vi "Autonomous Independent.vi"() -> ()   [LabVIEW 2012]
doc: "This VI is called when autonomous begins, and will automatically be terminated when autonomous ends. You can carry out timed or sensor driven robot movement independently without needing to return to the caller."
uses:
  Robot Global Data.vi
panel:
  out "Current Movement, for debugging":T1 {"Y Joystick Value" scale=1.0..-1.0; "X Joystick Value" scale=-1.0..1.0}
  in  "Array of robot movements":T2(array[cluster]) {"Y Joystick Value" scale=1.0..-1.0; "X Joystick Value" scale=-1.0..1.0}
  # "Be sure to right-click and choose Data Operations>>Make Current Value default if you want to save the array values with the VI"
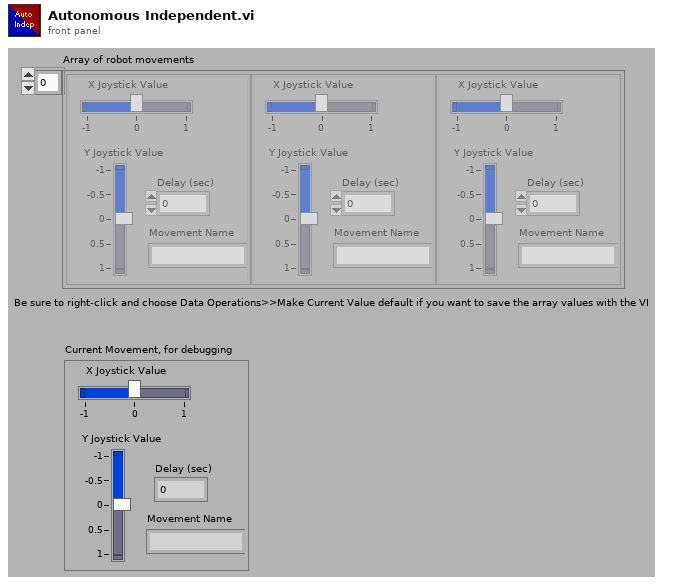
[diagram p1: front panel]
types:
  T1 = cluster{"X Joystick Value":dbl, "Y Joystick Value":dbl, "Delay (sec)":dbl, "Movement Name":string}
  T2 = cluster{"X Joystick Value":dbl, "Y Joystick Value":dbl, "Delay (sec)":dbl, "Movement Name":string}[]
  T3 = typedef "WPI_JoystickDevRef.ctl" = cluster{"Device":T4}
  T4 = typedef "WPI_JoystickDeviceEnum.ctl" = enum16{"USB 1", "USB 2", "USB 3", "USB 4", "Kinect 1", "Kinect 2"}
  T5 = cluster{"axis 1 (x)":dbl, "axis 2 (y)":dbl, "axis 3 (throttle)":dbl, "axis 4":dbl, "axis 5":dbl, "axis 6":dbl}
  T6 = typedef "WPI_DigitalInputDevRef.ctl" = cluster{"DevStatus":errorcluster, "DIO Channel":T7, "Digital Module":T8}
  T7 = typedef "FPGA_DIOChannel.ctl" = enum8{"DIO 1", "DIO 2", "DIO 3", "DIO 4", "DIO 5", "DIO 6", "DIO 7", "DIO 8", "DIO 9", "DIO 10", "DIO 11", "DIO 12", "DIO 13", "DIO 14", "Invalid"}
  T8 = typedef "FPGA_TypedefDigitalModule.ctl" = enum16{"Digital Module 1", "Digital Module 2"}
  T9 = typedef "WPI_RobotDriveDevRef.ctl" = cluster{"DevStatus":errorcluster, "Motors[]":T10[], "Square Inputs":bool, "Max Output":dbl, "Isochronous":bool}
  T10 = typedef "WPI_MotorControlDeviceRef.ctl" = cluster{"DeviceStatus":errorcluster, "Type":enum16{"PWM", "CAN"}, "PWM":cluster{"Digital Module":T8, "PWM Channel":T11, "DeadBand":T12}, "CAN":cluster{"Device Number":u8, "Control Mode":T13, "Semaphore":T14, "Max Vout":dbl}, "Invert":bool, "TransformRef":T15, "InvTransformRef":T15}
  T11 = typedef "FPGA_DIOPWMChannel.ctl" = enum8{"PWM 1", "PWM 2", "PWM 3", "PWM 4", "PWM 5", "PWM 6", "PWM 7", "PWM 8", "PWM 9", "PWM 10", "Invalid"}
  T12 = typedef "WPI_PWMDeadband.ctl" = cluster{"Name":string, "maxPositivePwm":i32, "minPositivePwm":i32, "centerPwm":i32, "maxNegativePwm":i32, "minNegativePwm":i32, "angularRange":u16}
  T13 = typedef "WPI_CANJaguar_ControlMode.ctl" = enum8{"Percent VBus", "Current", "Speed", "Position", "Voltage"}
  T14 = typedef "Semaphore RefNum" = refnum<k1>
  T15 = typedef "WPI_PWMTransform_ConPane.ctl" = refnum<vi>
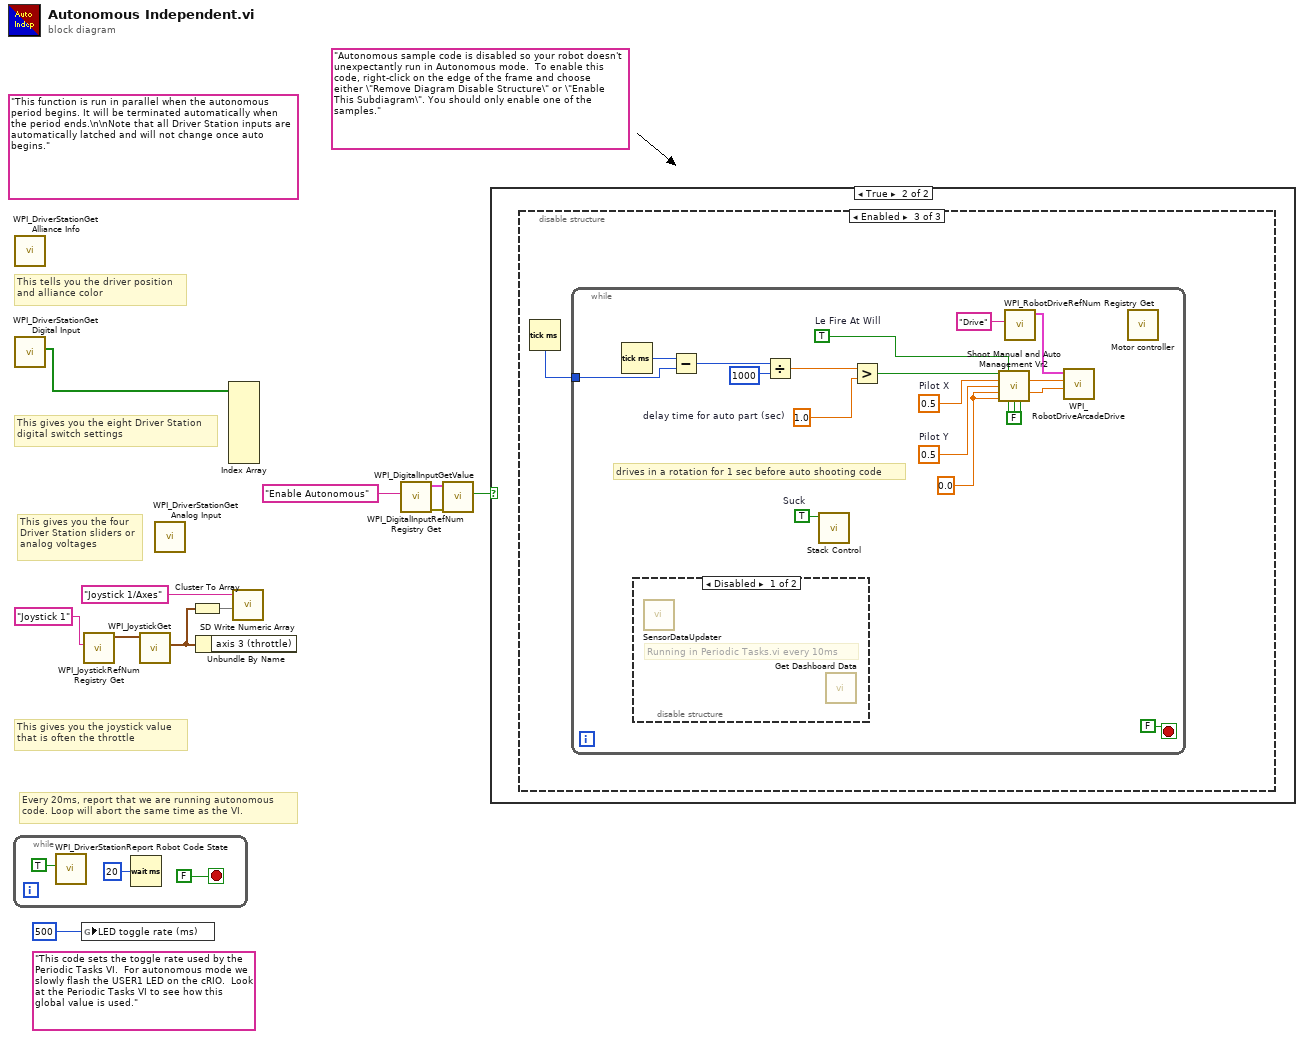
[diagram p0: block diagram]
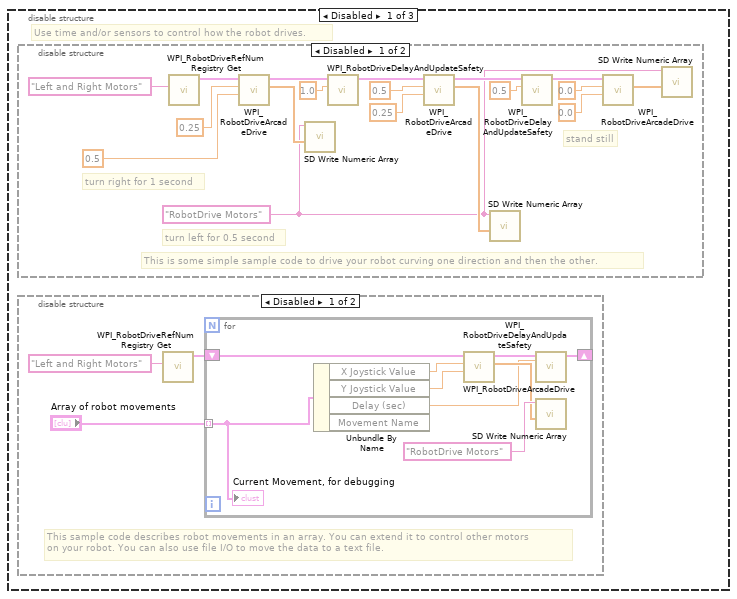
[diagram p3: hidden frame]
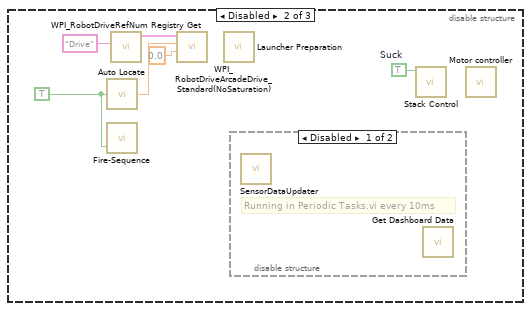
[diagram p6: hidden frame]
diagram:
  (unwired) "This code sets the toggle rate used by the Periodic Tasks VI.  For autonomous mode we slowly flash the USER1 LED on the cRIO.  Look at the Periodic Tasks VI to see how this global value is used."
  (unwired) "Autonomous sample code is disabled so your robot doesn't unexpectantly run in Autonomous mode.  To enable this code, right-click on the edge of the frame and choose either \"Remove Diagram Disable Structure\" or \"Enable This Subdiagram\". You should only enable one of the samples."
  (unwired) "This function is run in parallel when the autonomous period begins. It will be terminated automatically when the period ends.\n\nNote that all Driver Station inputs are automatically latched and will not change once auto begins."
  # "Every 20ms, report that we are running autonomous\ncode. Loop will abort the same time as the VI."
  # "This gives you the joystick value\nthat is often the throttle"
  # "This tells you the driver position\nand alliance color"
  # "This gives you the eight Driver Station\ndigital switch settings"
  # "This gives you the four\nDriver Station sliders or\nanalog voltages"
  n1 = while {
    stop <- FALSE stop-if-true
    n2 = call <vilib>:"WPI_DriverStationReport Robot Code State.vi"("Autonomous"=TRUE) -> ()  [unwired: 10 in, 1 out]
    n3 = Wait (ms)(milliseconds to wait=u32 20) -> ()  [unwired: 1 out]
  }
  n4 = call <vilib>:"WPI_DriverStationGet Alliance Info.vi"() -> ()  [unwired: 12 out]
  n5 = call <vilib>:"WPI_DriverStationGet Digital Input.vi"() -> ("Driver Station Digital Input (1-8)"=w11:bool[])  [unwired: 11 out]
  n6 = global write "Robot Global Data.vi" "LED toggle rate (ms)"(u32 500 ("LED ms toggle rate")) -> ()
  n7 = call <vilib>:"WPI_JoystickRefNum Registry Get.vi"("refnum name"="Joystick 1") -> ("JoystickDevRef"=w9:T3)  [unwired: 1 in, 9 out]
  n8 = call <vilib>:"WPI_JoystickGet.vi"("JoystickDevRef"=w9) -> ("Axes"=w6:T5)  [unwired: 1 in, 5 out]
  n9 = call <vilib>:"WPI_DriverStationGet Analog Input.vi"() -> ()  [unwired: 12 out]
  n10 = Cluster To Array(cluster=w6) -> (array=w7:dbl[])
  n11 = Unbundle By Name(w6) -> ()  [unwired: 1 out]
  n12 = Index Array(array=w11) -> ()  [unwired: 8 in, 8 out]
  n13 = call <vilib>:"SD Write Numeric Array.vi"("Numeric Array"=w7, "Name"="Joystick 1/Axes") -> ()  [unwired: 8 in, 2 out]
  n14 = call <vilib>:"WPI_DigitalInputRefNum Registry Get.vi"("refnum name"="Enable Autonomous") -> ("error out"=w2:errorcluster, "DigitalInputDevRef"=w4:T6)  [unwired: 9 in]
  n15 = call <vilib>:"WPI_DigitalInputGetValue.vi"("error in (no error)"=w2, "DigitalInputDevRef"=w4) -> ("Value"=w1:bool)  [unwired: 7 in, 2 out]
  n16 = case shown="True" w1 {
    frame False {
    }
    frame True {
      n17 = disable-structure shown="Enabled" {
        frame Disabled {
          # "Use time and/or sensors to control how the robot drives."
          n18 = disable-structure shown="Disabled" {
            frame Disabled {
              w27 = "RobotDrive Motors" ("Name")
              # "This is some simple sample code to drive your robot curving one direction and then the other."
              # "stand still"
              # "turn left for 0.5 second"
              # "turn right for 1 second"
              n19 = call <vilib>:"WPI_RobotDriveRefNum Registry Get.vi"("refnum name"="Left and Right Motors") -> ("RobotDriveDevRef"=w31:T9)  [unwired: 1 in, 9 out]
              n20 = call-poly <vilib>:"WPI_RobotDriveArcadeDrive.vi"("Y axis value"=0.5 ("X axis value"), "X axis value"=0.25, "RobotDriveDevRef"=w31) -> ("Motor Values"=w30:dbl[], "RobotDriveDevRef"=w38:T9)  [unwired: 1 in, 6 out]
              n21 = call <vilib>:"SD Write Numeric Array.vi"("Numeric Array"=w30, "Name"=w27) -> ()  [unwired: 8 in, 2 out]
              n22 = call <vilib>:"WPI_RobotDriveDelayAndUpdateSafety.vi"("Delay (s)"=1.0, "RobotDriveDevRef"=w38) -> ("RobotDriveDevRef 2"=w37:T9)  [unwired: 8 in, 1 out]
              n23 = call-poly <vilib>:"WPI_RobotDriveArcadeDrive.vi"("Y axis value"=0.25 ("X axis value"), "X axis value"=0.5, "RobotDriveDevRef"=w37) -> ("Motor Values"=w29:dbl[], "RobotDriveDevRef"=w36:T9)  [unwired: 1 in, 6 out]
              n24 = call <vilib>:"SD Write Numeric Array.vi"("Numeric Array"=w29, "Name"=w27) -> ()  [unwired: 8 in, 2 out]
              n25 = call <vilib>:"WPI_RobotDriveDelayAndUpdateSafety.vi"("Delay (s)"=0.5, "RobotDriveDevRef"=w36) -> ("RobotDriveDevRef 2"=w35:T9)  [unwired: 8 in, 1 out]
              n26 = call-poly <vilib>:"WPI_RobotDriveArcadeDrive.vi"("Y axis value"=0.0 ("X axis value"), "X axis value"=0.0, "RobotDriveDevRef"=w35) -> ("Motor Values"=w28:dbl[])  [unwired: 1 in, 7 out]
              n27 = call <vilib>:"SD Write Numeric Array.vi"("Numeric Array"=w28, "Name"=w27) -> ()  [unwired: 8 in, 2 out]
            }
            frame Enabled {
            }
          }
          n28 = disable-structure shown="Disabled" {
            frame Disabled {
              # "This sample code describes robot movements in an array. You can extend it to control other motors\non your robot. You can also use file I/O to move the data to a text file."
              n29 = call <vilib>:"WPI_RobotDriveRefNum Registry Get.vi"("refnum name"="Left and Right Motors") -> ("RobotDriveDevRef"=w16:T9)  [unwired: 1 in, 9 out]
              n30 = for {
                shift-right: [w22] -> _
                shift-left: w16 -> [w23]
                tunnel: "Array of robot movements" -> [w18] mode=indexing
                n31 = Unbundle By Name(w18) -> ("X Joystick Value"=w21:dbl, "Y Joystick Value"=w20:dbl, "Delay (sec)"=w19:dbl)  [unwired: 1 out]
                n32 = call-poly <vilib>:"WPI_RobotDriveArcadeDrive.vi"("Y axis value"=w20, "X axis value"=w21, "RobotDriveDevRef"=w23) -> ("Motor Values"=w25:dbl[], "RobotDriveDevRef"=w24:T9)  [unwired: 1 in, 6 out]
                n33 = call <vilib>:"WPI_RobotDriveDelayAndUpdateSafety.vi"("Delay (s)"=w19, "RobotDriveDevRef"=w24) -> ("RobotDriveDevRef 2"=w22:T9)  [unwired: 8 in, 1 out]
                n34 = call <vilib>:"SD Write Numeric Array.vi"("Numeric Array"=w25, "Name"="RobotDrive Motors") -> ()  [unwired: 8 in, 2 out]
                "Current Movement, for debugging" <- w18
              }
            }
            frame Enabled {
            }
          }
        }
        frame Disabled {
          w45 = TRUE  # Suck
          w47 = TRUE
          n35 = call "Auto Locate.vi"("Autonomous?"=w47) -> ("X Drive Arcade"=w46:dbl)
          n36 = call "Fire-Sequence.vi"("La Fire at will?"=w47) -> ()  [unwired: 3 in]
          n37 = call <vilib>:"WPI_RobotDriveRefNum Registry Get.vi"("refnum name"="Drive") -> ("RobotDriveDevRef"=w49:T9)  [unwired: 1 in, 9 out]
          n38 = call <vilib>:"WPI_RobotDriveArcadeDrive_Standard(NoSaturation).vi"("Y axis value"=0.0, "X axis value"=w46, "RobotDriveDevRef"=w49) -> ()  [unwired: 1 in, 8 out]
          n39 = call "Launcher Preparation.vi"() -> ()  [unwired: 5 in]
          n40 = disable-structure shown="Disabled" {
            frame Disabled {
              # "Running in Periodic Tasks.vi every 10ms"
              n41 = call "SensorDataUpdater.vi"() -> ()  [unwired: 12 in]
              n42 = call "Get Dashboard Data.vi"() -> ()  [unwired: 12 in]
            }
            frame Enabled {
            }
          }
          n43 = call "Stack Control.vi"("Suck"=w45) -> ()  [unwired: 4 in, 7 out]
          n44 = call "Motor controller.vi"() -> ()  [unwired: 12 in]
        }
        frame Enabled {
          n45 = Tick Count (ms)() -> (millisecond timer value=w51:u32)
          n46 = while {
            tunnel: w51 -> [w63]
            stop <- FALSE stop-if-true
            w52 = TRUE  # Suck
            w53 = FALSE
            w55 = 0.0 ("Elevation")
            w56 = 0.5  # Pilot Y
            w58 = 1.0  # delay time for auto part (sec)
            w60 = 0.5  # Pilot X
            w69 = TRUE  # Le Fire At Will
            # "drives in a rotation for 1 sec before auto shooting code"
            n47 = Tick Count (ms)() -> (millisecond timer value=w64:u32)
            n48 = disable-structure shown="Disabled" {
              frame Disabled {
                # "Running in Periodic Tasks.vi every 10ms"
                n49 = call "SensorDataUpdater.vi"() -> ()  [unwired: 12 in]
                n50 = call "Get Dashboard Data.vi"() -> ()  [unwired: 12 in]
              }
              frame Enabled {
              }
            }
            n51 = Subtract(x=w64, y=w63) -> (x-y=w62:u32)
            n52 = Divide(x=w62, y=u32 1000) -> (x/y=w59:dbl)
            n53 = call "Stack Control.vi"("Suck"=w52) -> ()  [unwired: 4 in, 7 out]
            n54 = Greater?(x=w59, y=w58) -> (0:w57:bool)
            n55 = call "Shoot Manual and Auto Management Vr2.vi"("Auto Preparation for Shooting"=w57, "Le Fire At Will"=w69, "Pilot X"=w60, "Pilot Y"=w56, "Elevation"=w55, "Shoot Motors"=w55, "Stop Centerizing"=w53, "ReCenterize"=w53, "Fine Tune"=w53) -> ("X Drive Arcade"=w67:dbl, "Y Drive Arcade"=w66:dbl)  [unwired: 4 in, 1 out]
            n56 = call <vilib>:"WPI_RobotDriveRefNum Registry Get.vi"("refnum name"="Drive") -> ("RobotDriveDevRef"=w65:T9)  [unwired: 9 in, 1 out]
            n57 = call-poly <vilib>:"WPI_RobotDriveArcadeDrive.vi"("Y axis value"=w66, "X axis value"=w67, "RobotDriveDevRef"=w65) -> ()  [unwired: 6 in, 3 out]
            n58 = call "Motor controller.vi"() -> ()  [unwired: 12 in]
          }
        }
      }
    }
  }
